vi "getWriteFile.vi"(0 "refnum in":refnum<file>, 1 "from (0:start)":enum16{"start", "end", "current"}(ring), 2 "offset (in bytes) (0)":i64, 3 "error in":errorcluster, 4 "Data":string[][](array[string])) -> (5 "refnum out":refnum<file>, 6 "position after write(bytes)":i32, 7 "error out":errorcluster)   [LabVIEW 2017]
uses:
  <vilib>/Utility/file.llb/Write Delimited Spreadsheet (string).vi
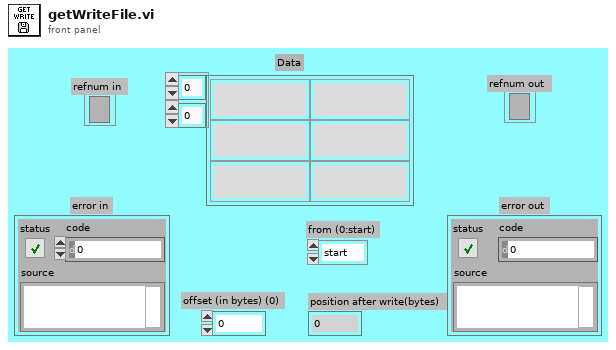
[diagram p1: front panel]
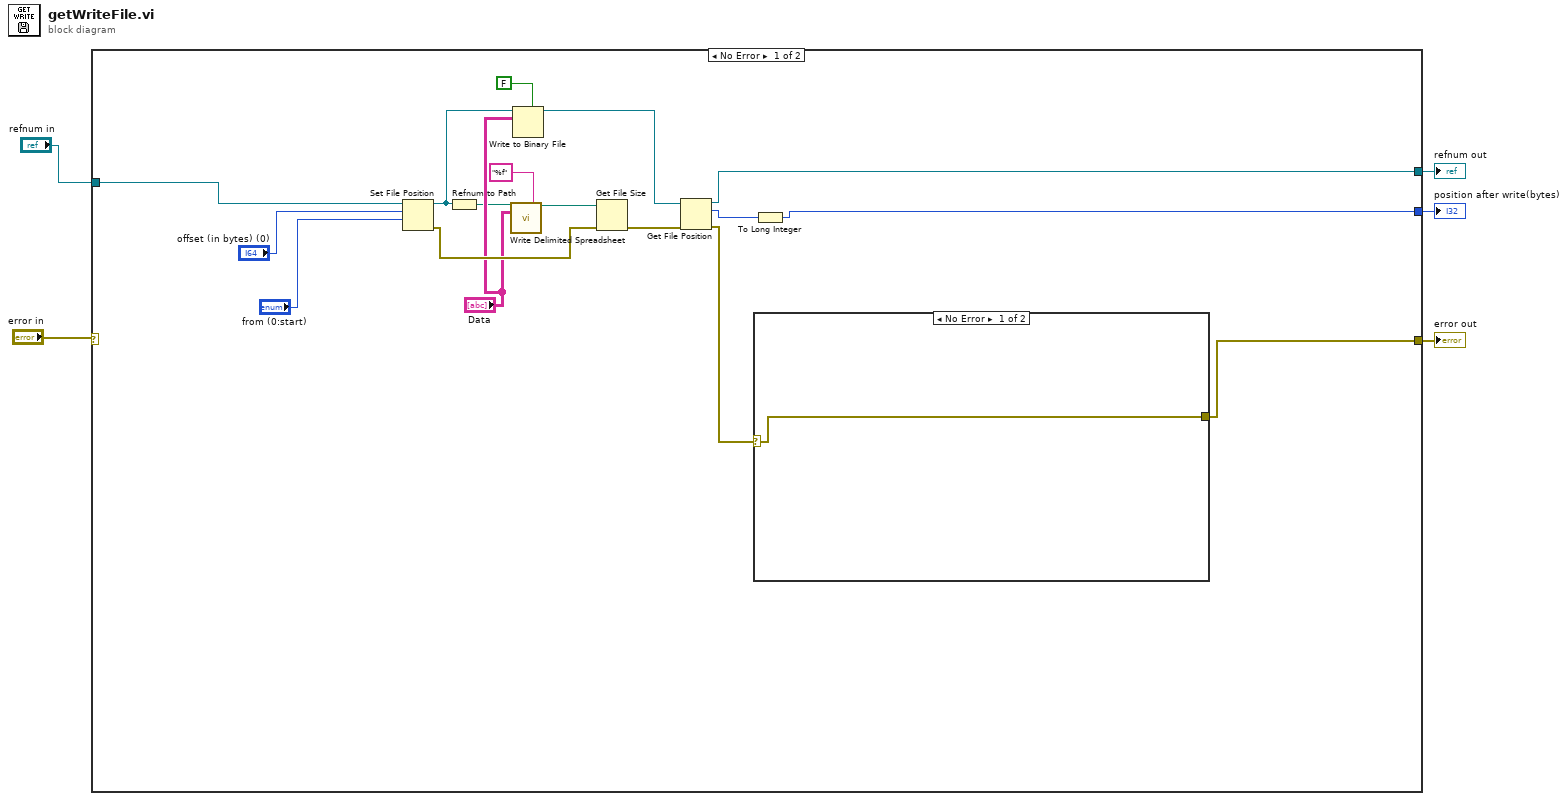
[diagram p0: block diagram]
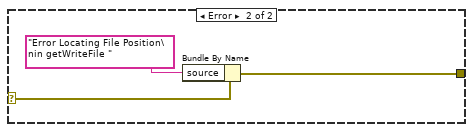
[diagram p2: hidden frame]
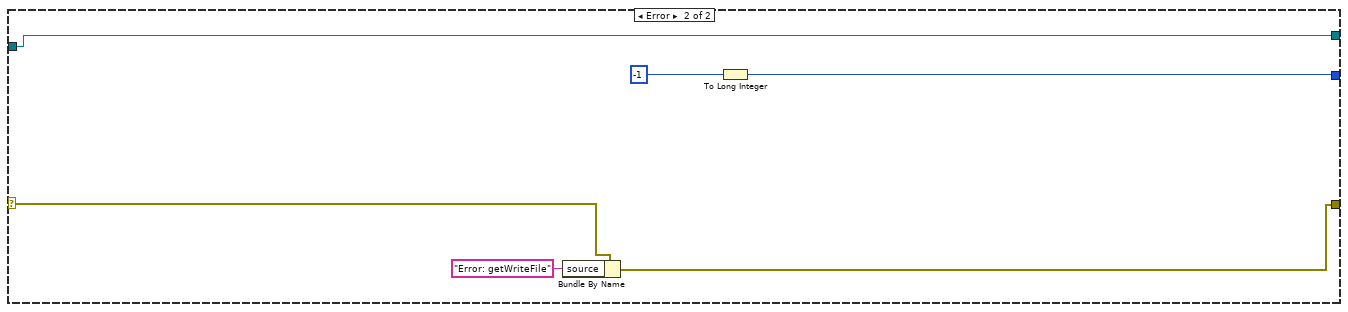
[diagram p3: hidden frame]
diagram:
  n1 = case shown="No Error" "error in" {
    selector: "error in" -> [_ w29]
    tunnel: "refnum in" -> [w19 w32]
    tunnel: [w17 w27] -> w1
    tunnel: [w16 w30] -> w2
    tunnel: [w15 w32] -> w3
    frame No Error {
      n2 = Set File Position(offset (in bytes) (0)="offset (in bytes) (0)", refnum=w19, from (0:start)="from (0:start)") -> (refnum out=w10:refnum<file>, error out=w13:errorcluster)  [unwired: 1 in]
      n3 = Refnum to Path(1:w10) -> (0:w6:path)
      n4 = call-poly <vilib>:"Write Delimited Spreadsheet.vi"("file path (dialog if empty)"=w6, "format (%s)"="%f", "2D data"="Data") -> ("new file path (Not A Path if cancelled)"=w14:path)  [unwired: 11 in, 1 out]
      n5 = Write to Binary File(file (use dialog)=w10, data="Data", 5:FALSE ("prepend array or string size? (T)")) -> (refnum out=w7:refnum<file>)  [unwired: 3 in, 2 out]
      n6 = Get File Size(file=w14, error in=w13) -> (0:w12:errorcluster)  [unwired: 2 out]
      n7 = Get File Position(4:w12, 7:w7) -> (0:w18:errorcluster, 2:w20:i64, 3:w15:refnum<file>)
      n8 = case shown="No Error" w18 {
        selector: w18 -> [w23 w26]
        tunnel: [w23 w24] -> w17
        frame No Error {
        }
        frame Error {
          n9 = Bundle By Name(cluster=w26, "source"="Error Locating File Position\nin getWriteFile ") -> (w24:errorcluster)
        }
      }
      n10 = To Long Integer(number=w20) -> (32bit integer=w16:i32)
    }
    frame Error {
      n11 = Bundle By Name(cluster=w29, "source"="Error: getWriteFile") -> (w27:errorcluster)
      n12 = To Long Integer(number=-1) -> (32bit integer=w30:i32)
    }
  }
  "refnum out" <- w3
  "position after write(bytes)" <- w2
  "error out" <- w1
